vi "simulate-robot.vi"() -> ()   [LabVIEW 2019]
uses:
  ROBOT_PICTURE.ctl
  <vilib>/Rock Robotics/WPI/Camera/WPI_CameraImageSize.ctl
  <vilib>/Rock Robotics/WPI/ThirdParty/JAS_Junk/TrajLib/Transform_Create_PosePose.vi
  <vilib>/Rock Robotics/WPI/ThirdParty/JAS_Junk/TrajLib/Util_CalcDist.vi
  <vilib>/Rock Robotics/WPI/ThirdParty/JAS_Junk/TrajLib/Rotation_UnaryMinus.vi
  <vilib>/Rock Robotics/WPI/ThirdParty/JAS_Junk/TrajLib/Translation_RotateBy.vi
  <vilib>/Rock Robotics/WPI/ThirdParty/JAS_Junk/TrajLib/Translation_Minus.vi
  <vilib>/Rock Robotics/WPI/ThirdParty/JAS_Junk/TrajLib/Rotation_Minus.vi
  <vilib>/Rock Robotics/WPI/ThirdParty/JAS_Junk/TrajLib/Rotation_RotateBy.vi
  Robot Global Data.vi
  <vilib>/Rock Robotics/WPI/ThirdParty/JAS_Junk/TrajLib/Trajectory_Library.lvlib
panel:
  in  "Finish":bool
  in  "Enable Vision":bool
  in  "Image Size":T1=enum."320x240"
  out "BALL":bool=TRUE
  in  "Y  INCHES - BALL":dbl=150.0
  in  "X INCHES - BALL":dbl=150.0
  out "2D Picture":T2
  # "BALL"
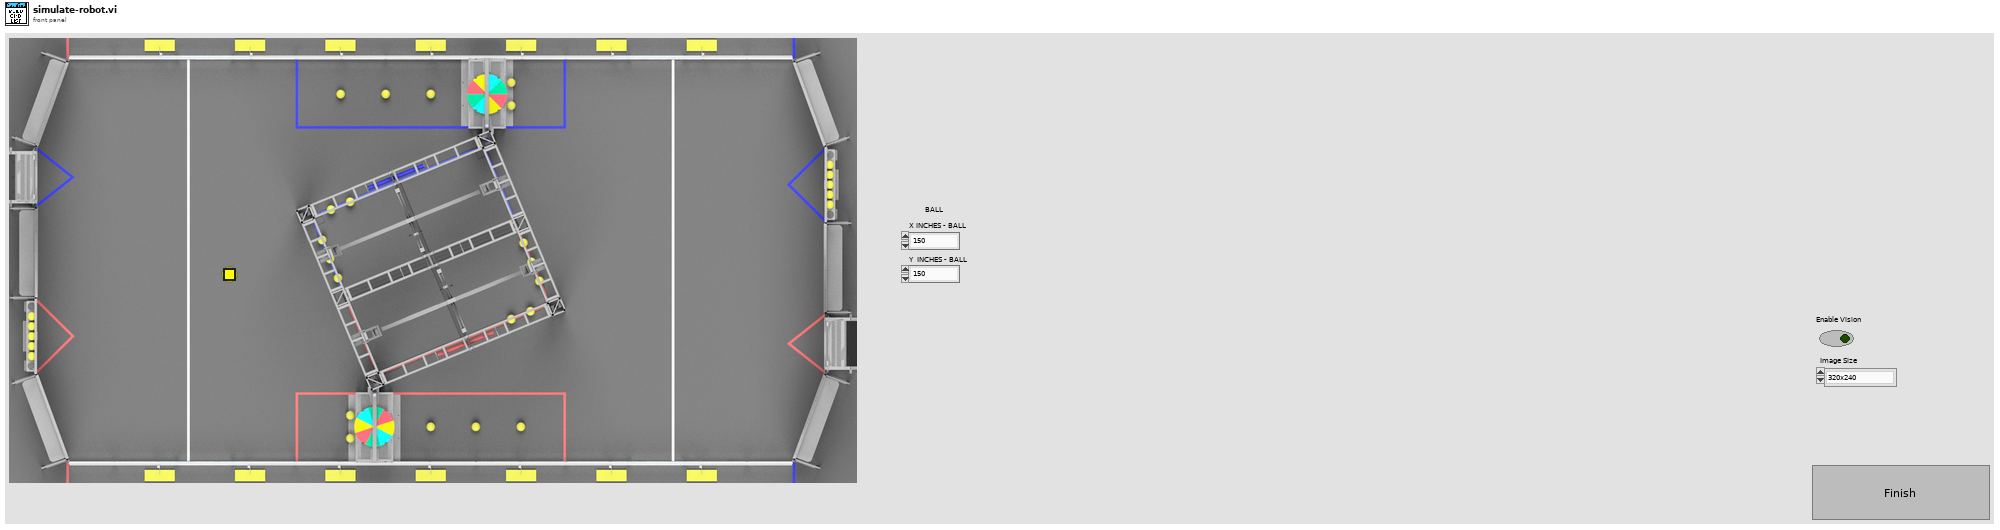
[diagram p1: front panel]
types:
  T1 = typedef "WPI_CameraImageSize.ctl" = enum16{"640x480", "320x240", "160x120", "Custom"}
  T2 = typedef "ROBOT_PICTURE.ctl" = picture
  T3 = typedef "WPI_DriverStationMatch Info.ctl" = cluster{"Autonomous Elapsed Seconds":dbl, "TeleOp Elapsed Seconds":dbl, "Disabled Elapsed Seconds":dbl, "Visited Autonomous":bool, "Visited TeleOp":bool, "Visited Disabled":bool, "Autonomous Settings":cluster{"Autonomous Style":enum16{"Iterative", "Independent"}, "VI Refnum":refnum<vi>}}
  T4 = typedef "WPI_DriverStationDerivedRobotMode.ctl" = enum16{"Init", "Execute", "Stop"}
  T5 = typedef "WPI_DriverStationRobotMode2.ctl" = enum16{"Autonomous Disabled", "Autonomous Enabled", "Teleop Disabled", "Teleop Enabled", "Disconnected", "Finish", "Test Disabled", "Test Enabled", "Emergency Stopped"}
  T6 = typedef "imagedata.ctl" = cluster{"image type":i32, "image depth":i32, "image":u8[], "mask":u8[], "colors":u32[], "Rectangle":cluster{"left":i16, "top":i16, "right":i16, "bottom":i16}}
  T7 = typedef "Trajectory_Library.lvlib/SWERVE_DRIVE_ODOMETRY.ctl" = cluster{"POSE":T8, "GyroOffset":T10, "PreviousAngle":T10, "PrevTime":dbl}
  T8 = typedef "Trajectory_Library.lvlib/POSE2D.ctl" = cluster{"TRANSLATION":T9, "ROTATION":T10}
  T9 = typedef "Trajectory_Library.lvlib/TRANSLATION2D.ctl" = cluster{"X":dbl, "Y":dbl}
  T10 = typedef "Trajectory_Library.lvlib/ROTATION2D.ctl" = cluster{"VALUE":dbl, "COS":dbl, "SIN":dbl}
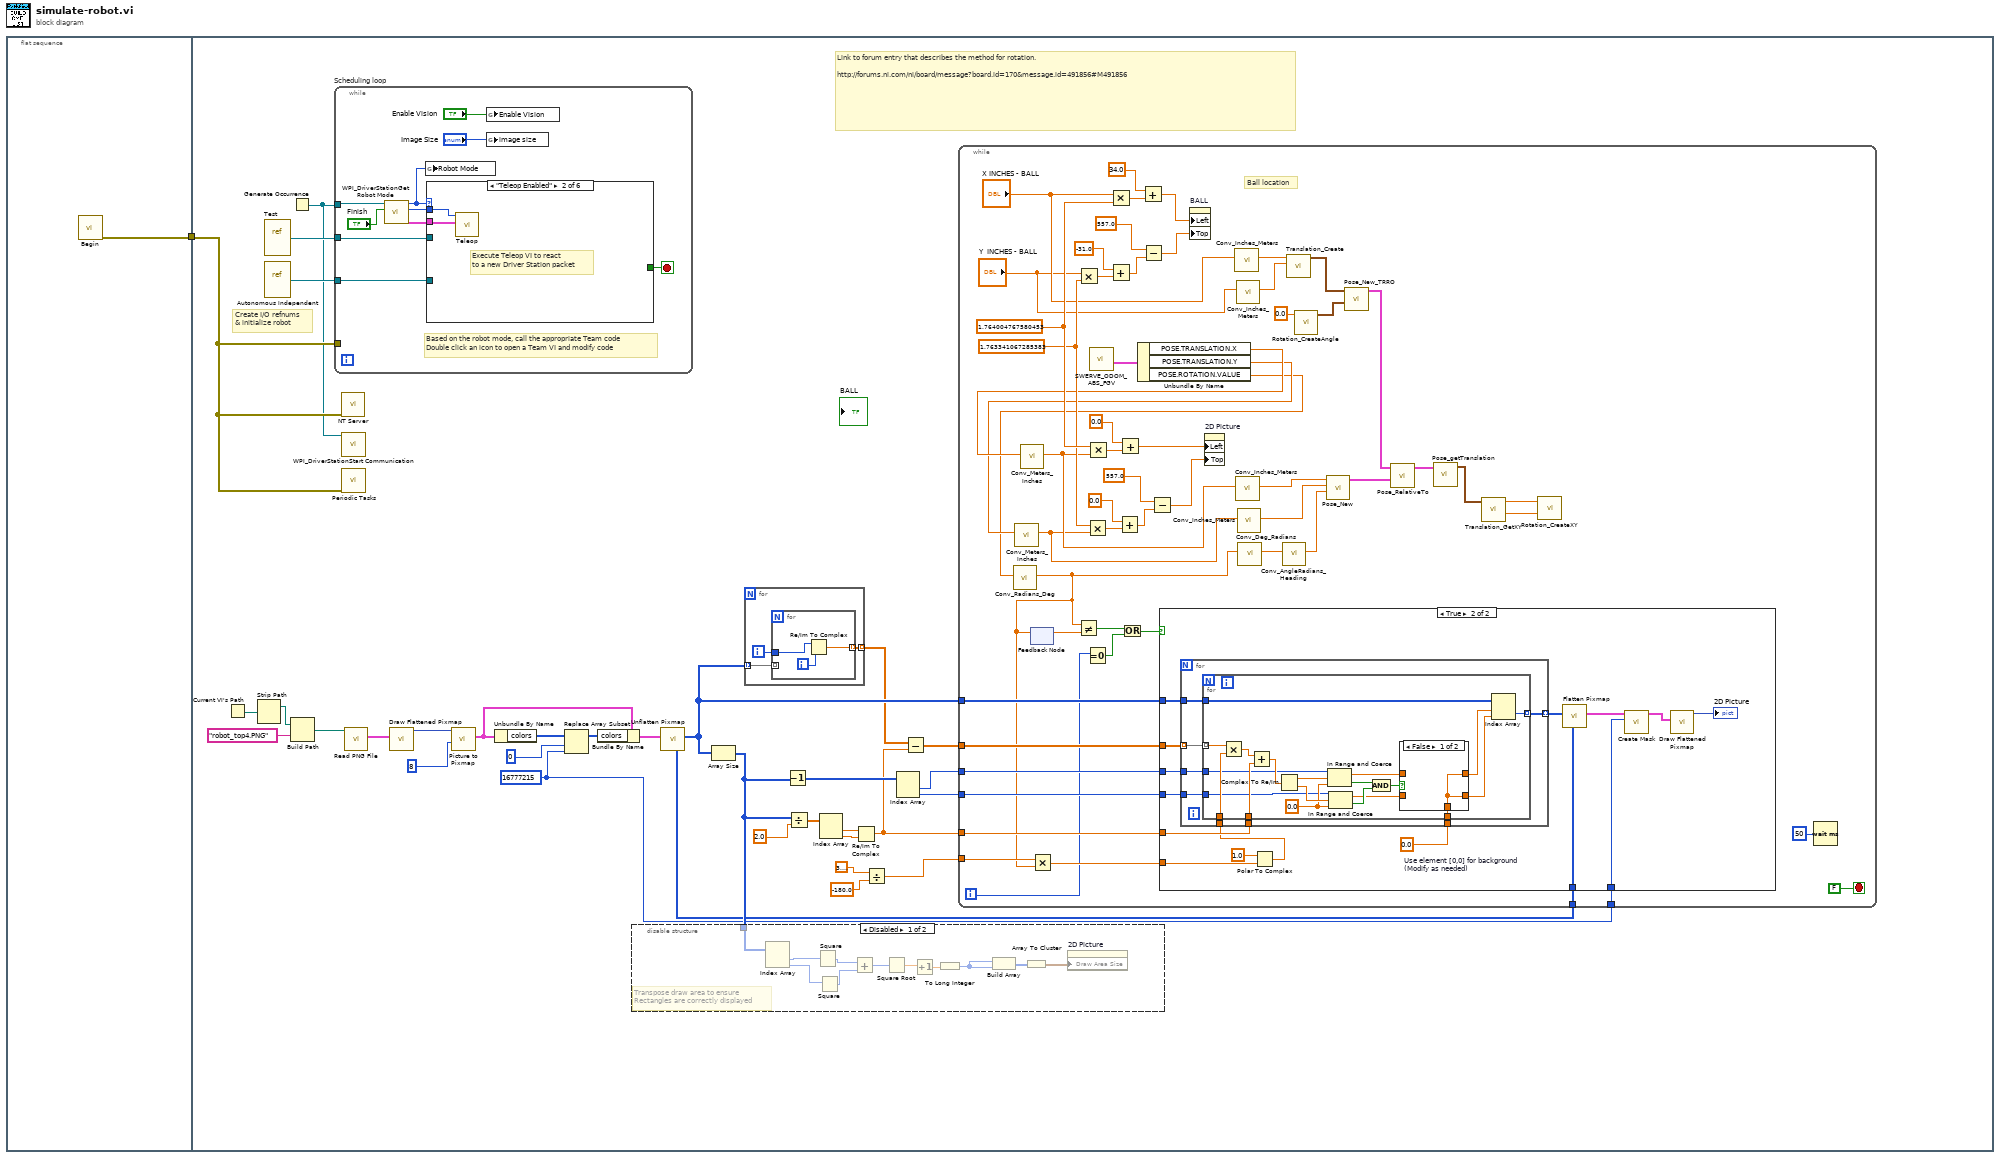
[diagram p0: block diagram]
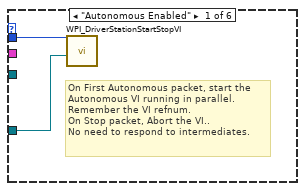
[diagram p2: hidden frame]
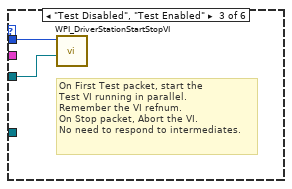
[diagram p3: hidden frame]
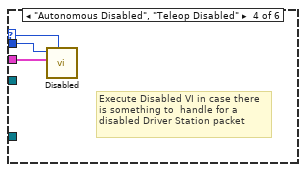
[diagram p4: hidden frame]
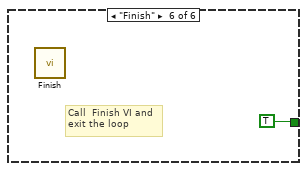
[diagram p6: hidden frame]
diagram:
  n1 = flat-sequence {
    tunnel: [w2] -> w1
    tunnel: w1 -> [w4]
    frame #0 {
      n2 = call "Begin.vi"() -> ("error out"=w2:errorcluster)  [unwired: 11 in]
    }
    frame #1 {
      w12 = u32 16777215 ("new element/subarray")
      # "Create I/O refnums\n& initialize robot"
      # "Link to forum entry that describes the method for rotation.\n\nhttp://forums.ni.com/ni/board/message?board.id=170&message.id=491856#M491856"
      n3 = Current VI's Path() -> (path=w25:path)
      n4 = Strip Path(path=w25) -> (stripped path=w27:path)  [unwired: 1 out]
      n5 = vi-ref "Test.vi"() -> (w5:refnum<vi>)
      n6 = vi-ref "Autonomous Independent.vi"() -> (w6:refnum<vi>)
      n7 = Generate Occurrence() -> (w3:refnum<k4>)
      n8 = Build Path(base path=w27, name or relative path="robot_top4.PNG") -> (appended path=w26:path)
      n9 = while "Scheduling loop" {
        tunnel: w3 -> [w44]
        tunnel: w4 -> [_]
        tunnel: w6 -> [w39]
        tunnel: w5 -> [w37]
        stop <- w41 stop-if-true
        # "Based on the robot mode, call the appropriate Team code\nDouble click an icon to open a Team VI and modify code"
        n10 = call <vilib>:"WPI_DriverStationGet Robot Mode.vi"("Finish"="Finish", "DS Occurrence"=w44) -> ("Match Info out"=w42:T3, "Call Context"=w45:T4, "Robot Mode"=w36:T5)  [unwired: 7 out]
        n11 = global write "Robot Global Data.vi" "Robot Mode"(w36) -> ()
        n12 = case shown="\"Teleop Enabled\"" w36 {
          selector: w36 -> [_ _ _ w52 _ _]
          tunnel: w45 -> [w47 w49 w51 w54 _ _]
          tunnel: w42 -> [_ w48 _ w53 _ _]
          tunnel: [_ _ _ _ _ TRUE] -> w41
          tunnel: w39 -> [w46 _ _ _ _ _]
          tunnel: w37 -> [_ _ w50 _ _ _]
          frame "Autonomous Enabled" {
            # "On First Autonomous packet, start the\nAutonomous VI running in parallel.\nRemember the VI refnum.\nOn Stop packet, Abort the VI..\nNo need to respond to intermediates."
            n13 = call <vilib>:"WPI_DriverStationStartStopVI.vi"("VI in"=w46, "Call Context"=w47) -> ()  [unwired: 10 in]
          }
          frame "Teleop Enabled" {
            # "Execute Teleop VI to react\nto a new Driver Station packet"
            n14 = call "Teleop.vi"("Match Info"=w48, "Call Context"=w49) -> ()  [unwired: 1 in, 9 out]
          }
          frame "Test Disabled", "Test Enabled" {
            # "On First Test packet, start the\nTest VI running in parallel.\nRemember the VI refnum.\nOn Stop packet, Abort the VI.\nNo need to respond to intermediates."
            n15 = call <vilib>:"WPI_DriverStationStartStopVI.vi"("VI in"=w50, "Call Context"=w51) -> ()  [unwired: 10 in]
          }
          frame "Autonomous Disabled", "Teleop Disabled" {
            # "Execute Disabled VI in case there\nis something to  handle for a\ndisabled Driver Station packet"
            n16 = call "Disabled.vi"("Robot Mode"=w52, "Match Info"=w53, "Call Context"=w54) -> ()  [unwired: 1 in, 8 out]
          }
          frame "Disconnected", Default {
            # "Driver Station packet didn't arrive.\nPossibly useful for diagnostics"
          }
          frame "Finish" {
            # "Call  Finish VI and\nexit the loop"
            n17 = call "Finish.vi"() -> ()  [unwired: 1 in, 7 out]
          }
        }
        n18 = global write "Robot Global Data.vi" "Enable Vision"("Enable Vision") -> ()
        n19 = global write "Robot Global Data.vi" "image size"("Image Size") -> ()
      }
      n20 = call <vilib>:"NT Server.vi"("error in (no error)"=w4) -> ()  [unwired: 11 in]
      n21 = call <vilib>:"WPI_DriverStationStart Communication.vi"("occurrence"=w3) -> ()  [unwired: 1 in, 10 out]
      n22 = call "Periodic Tasks.vi"("error in"=w4) -> ()  [unwired: 11 in]
      n23 = call <vilib>:"Read PNG File.vi"("path to PNG file"=w26) -> ("image data"=w32:T6)  [unwired: 8 in, 2 out]
      n24 = call <vilib>:"Draw Flattened Pixmap.vi"("image data"=w32) -> ("new picture"=w33:picture)  [unwired: 8 in]
      n25 = call <vilib>:"Picture to Pixmap.vi"("depth"=8, "picture"=w33) -> ("image data"=w34:T6)  [unwired: 8 in, 1 out]
      n26 = Unbundle By Name(w34) -> ("colors"=w30:u32[])
      n27 = Replace Array Subset(array=w30, new element=w12, index=0) -> (w31:u32[])
      n28 = Bundle By Name(cluster=w34, "colors"=w31) -> (w35:T6)
      n29 = call <vilib>:"Unflatten Pixmap.vi"("image data"=w35) -> ("8-bit pixmap"=w29:u8[][], "colors"=w18:u32[])  [unwired: 4 in, 5 out]
      n30 = Array Size(array=w29) -> (size(s)=w28:i32[])
      n31 = disable-structure shown="Disabled" {
        disable-tunnel: w28 -> [w66 _]
        frame Disabled {
          # "Transpose draw area to ensure \nRectangles are correctly displayed"
          n32 = Index Array(array=w66) -> (element #1=w65:i32, element #2=w64:i32)  [unwired: 2 in]
          n33 = Square(x=w65) -> (x^2=w63:i32)
          n34 = Square(x=w64) -> (x^2=w62:i32)
          n35 = Add(x=w63, y=w62) -> (x+y=w61:i32)
          n36 = Square Root(x=w61) -> (sqrt(x)=w60:dbl)
          n37 = Increment(x=w60) -> (x+1=w59:dbl)
          n38 = To Long Integer(number=w59) -> (32bit integer=w58:i32)
          n39 = Build Array(w58, w58) -> (w57:i32[])
          n40 = Array To Cluster(array=w57) -> (cluster=w56:cluster{"[0]":i32, "[1]":i32})
          n41 = property on="2D Picture" class="Pict (strict)"("Draw Area Size"=w56) -> ()  [unwired: 2 in, 2 out]
        }
        frame Enabled {
        }
      }
      n42 = for {
        tunnel: [w172] -> w14 mode=indexing
        tunnel: w29 -> [w171] mode=indexing
        i -> [w173]
        n43 = for {
          tunnel: w173 -> [w176]
          tunnel: [w175] -> w172 mode=indexing
          tunnel: w171 -> [_] mode=indexing
          i -> [w174]
          n44 = Re/Im To Complex(1:w174, 2:w176) -> (0:w175:cdb)
        }
      }
      n45 = Decrement(x=w28) -> (x-1=w24:i32[])
      n46 = Divide(x=w28, y=2.0) -> (x/y=w17:dbl[])
      n47 = Index Array(array=w17) -> (element #1=w20:dbl, element #2=w21:dbl)  [unwired: 2 in]
      n48 = Re/Im To Complex(1:w21, 2:w20) -> (0:w16:cdb)
      n49 = Divide(x=3.141592653589793, y=-180.0 ("value")) -> (x/y=w19:dbl)
      n50 = Index Array(array=w24) -> (element #1=w22:i32, element #2=w23:i32)  [unwired: 2 in]
      n51 = Subtract(x=w14, y=w16) -> (x-y=w15:cdb[][])
      n52 = while {
        tunnel: w29 -> [w124]
        tunnel: w15 -> [w123]
        tunnel: w16 -> [w122]
        tunnel: w18 -> [w121]
        tunnel: w19 -> [w120]
        tunnel: w22 -> [w119]
        tunnel: w23 -> [w118]
        tunnel: w12 -> [w114]
        i -> [w74]
        stop <- FALSE stop-if-true
        w95 = 1.763341067285383
        w102 = 1.764004767580453
        # "Ball location"
        n53 = feedback #1() -> (w113:dbl)  [unwired: 1 in]
        n54 = Multiply(x="Y  INCHES - BALL", y=w95) -> (x*y=w100:dbl)
        n55 = Equal To 0?(x=w74) -> (x = 0?=w75:bool)
        n56 = call "SWERVE_ODOM_ABS_FGV.vi"() -> ("out SWERVE_DRIVE_ODOMETRY"=w73:T7)  [unwired: 11 in]
        n57 = Multiply(x="X INCHES - BALL", y=w102) -> (x*y=w104:dbl)
        n58 = Add(x=-31.0, y=w100) -> (x+y=w97:dbl)
        n59 = Unbundle By Name(w73) -> ("POSE.TRANSLATION.X"=w71:dbl, "POSE.TRANSLATION.Y"=w69:dbl, "POSE.ROTATION.VALUE"=w67:dbl)
        n60 = call <vilib>:"Conv_Radians_Deg.vi"("Radians"=w67) -> ("Degrees"=w68:dbl)  [unwired: 10 in]
        n61 = call <vilib>:"Conv_Meters_Inches.vi"("Meters"=w69) -> ("Inches"=w70:dbl)  [unwired: 10 in]
        n62 = call <vilib>:"Conv_Meters_Inches.vi"("Meters"=w71) -> ("Inches"=w72:dbl)  [unwired: 10 in]
        n63 = feedback-in #1(w68) -> ()
        n64 = Multiply(x=w120, y=w68) -> (x*y=w116:dbl)
        n65 = Not Equal?(x=w68, y=w113) -> (x != y?=w76:bool)
        n66 = Multiply(x=w95, y=w70) -> (x*y=w110:dbl)
        n67 = Multiply(x=w102, y=w72) -> (x*y=w112:dbl)
        n68 = Add(x=0.0, y=w110) -> (x+y=w106:dbl)
        n69 = Add(x=0.0, y=w112) -> (x+y=w107:dbl)
        n70 = Or(x=w76, y=w75) -> (x .or. y?=w77:bool)
        n71 = Add(x=34.0, y=w104) -> (x+y=w101:dbl)
        n72 = Subtract(x=557.0, y=w97) -> (x-y=w96:dbl)
        n73 = Subtract(x=557.0, y=w106) -> (x-y=w105:dbl)
        n74 = case shown="True" w77 {
          tunnel: w124 -> [_ w139]
          tunnel: w123 -> [_ w138]
          tunnel: w122 -> [_ w137]
          tunnel: w121 -> [_ w136]
          tunnel: w119 -> [_ w135]
          tunnel: w118 -> [_ w134]
          tunnel: w116 -> [_ w131]
          tunnel: w114 -> [_ w125]
          frame False {
          }
          frame True {
            w130 = 0.0  # Use element [0,0] for background (Modify as needed)
            n75 = Polar To Complex(1:w131, 2:1.0 ("r")) -> (0:w129:cdb)
            n76 = for {
              tunnel: w129 -> [w147]
              tunnel: w139 -> [w146]
              tunnel: w137 -> [w145]
              tunnel: w138 -> [w144] mode=indexing
              tunnel: [w143] -> w133 mode=indexing
              tunnel: w130 -> [w142]
              tunnel: w135 -> [w141]
              tunnel: w134 -> [w140]
              n77 = for {
                tunnel: w146 -> [w167]
                tunnel: w147 -> [w162]
                tunnel: [w166] -> w143 mode=indexing
                tunnel: w145 -> [w164]
                tunnel: w144 -> [w161] mode=indexing
                tunnel: w142 -> [w148]
                tunnel: w141 -> [w156]
                tunnel: w140 -> [w155]
                w157 = 0.0 ("lower limit")
                n78 = Multiply(x=w161, y=w162) -> (x*y=w163:cdb)
                n79 = Add(x=w163, y=w164) -> (x+y=w165:cdb)
                n80 = Complex To Re/Im(x + iy=w165) -> (x=w160:dbl, y=w159:dbl)
                n81 = In Range and Coerce(upper limit=w156, x=w160, lower limit=w157) -> (coerced(x)=w151:dbl, In Range?=w158:bool)
                n82 = In Range and Coerce(upper limit=w155, x=w159, lower limit=w157) -> (coerced(x)=w149:dbl, In Range?=w154:bool)
                n83 = And(x=w158, y=w154) -> (x .and. y?=w153:bool)
                n84 = case shown="False" w153 {
                  tunnel: [w168 w170] -> w152
                  tunnel: w151 -> [_ w170]
                  tunnel: [w168 w169] -> w150
                  tunnel: w149 -> [_ w169]
                  tunnel: w148 -> [w168 _]
                  frame False {
                  }
                  frame True {
                  }
                }
                n85 = Index Array(array=w167, index (row)=w152, index (col)=w150) -> (element=w166:u8)
              }
            }
            n86 = call <vilib>:"Flatten Pixmap.vi"("colors"=w136, "8-bit pixmap"=w133) -> ("image data"=w127:T6)  [unwired: 9 in]
            n87 = call <vilib>:"Create Mask.vi"("Mask Color (Black)"=w125, "image data"=w127) -> ("image data"=w126:T6)  [unwired: 9 in]
            n88 = call <vilib>:"Draw Flattened Pixmap.vi"("image data"=w126) -> ("new picture"=→"2D Picture":picture)  [unwired: 8 in]
          }
        }
        n89 = property on="BALL" class="Bool (strict)"("Left"=w101, "Top"=w96) -> ()  [unwired: 2 in, 2 out]
        n90 = property on="2D Picture" class="Pict (strict)"("Left"=w107, "Top"=w105) -> ()  [unwired: 2 in, 2 out]
        n91 = call <vilib>:"Conv_Inches_Meters.vi"("INCH"="X INCHES - BALL") -> ("Meters"=w89:dbl)  [unwired: 10 in]
        n92 = call <vilib>:"Conv_Inches_Meters.vi"("INCH"=w72) -> ("Meters"=w93:dbl)  [unwired: 10 in]
        n93 = call <vilib>:"Conv_Inches_Meters.vi"("INCH"="Y  INCHES - BALL") -> ("Meters"=w88:dbl)  [unwired: 10 in]
        n94 = call <vilib>:"Conv_Inches_Meters.vi"("INCH"=w70) -> ("Meters"=w92:dbl)  [unwired: 10 in]
        n95 = call <vilib>:"Conv_Deg_Radians.vi"("Degress"=w68) -> ("Radians"=w94:dbl)  [unwired: 10 in]
        n96 = call <vilib>:"Conv_AngleRadians_Heading.vi"("Radians"=w94) -> ("Heading"=w85:dbl)  [unwired: 10 in]
        n97 = call <vilib>:"Translation_Create.vi"("Y"=w88, "X"=w89) -> ("TRANSLATION"=w87:T9)  [unwired: 9 in]
        n98 = call <vilib>:"Rotation_CreateAngle.vi"("Angle"=0.0) -> ("ROTATION"=w82:T10)  [unwired: 10 in]
        n99 = call <vilib>:"Pose_New.vi"("Heading"=w85, "Y"=w92, "X"=w93) -> ("out POSe"=w84:T8)  [unwired: 8 in]
        n100 = call <vilib>:"Pose_New_TRRO.vi"("ROTATION"=w82, "TRANSLATION"=w87) -> ("outPOSE"=w86:T8)  [unwired: 9 in]
        n101 = call <vilib>:"Pose_RelativeTo.vi"("other POSE"=w84, "in POSE"=w86) -> ("out POSE"=w81:T8)  [unwired: 9 in]
        n102 = call <vilib>:"Pose_getTranslation.vi"("in POSE"=w81) -> ("outTRANSLATION"=w80:T9)  [unwired: 10 in]
        n103 = call <vilib>:"Translation_GetXY.vi"("In Translation"=w80) -> ("Y"=w78:dbl, "X"=w79:dbl)  [unwired: 9 in]
        n104 = call <vilib>:"Rotation_CreateXY.vi"("Y or sine"=w78, "X or  cosine"=w79) -> ()  [unwired: 9 in, 1 out]
        n105 = Wait (ms)(milliseconds to wait=u32 50) -> ()  [unwired: 1 out]
      }
    }
  }
